vi "ConfigParseLoop.vi"(0 "Root Refnum in":refnum<k20>, 11 "error in (no error)":errorcluster) -> (4 "General Settings":string[][](array[string]), 6 "Loop Microscope Settings":string[][](array[string]), 8 "Position Settings":string[][](array[string]), 10 "Program":string[][](array[string]), 15 "error out":errorcluster)   [LabVIEW 2018, in "Config.lvlib"]
uses:
  Config.lvlib
  <vilib>/xml/NI_XML.lvlib
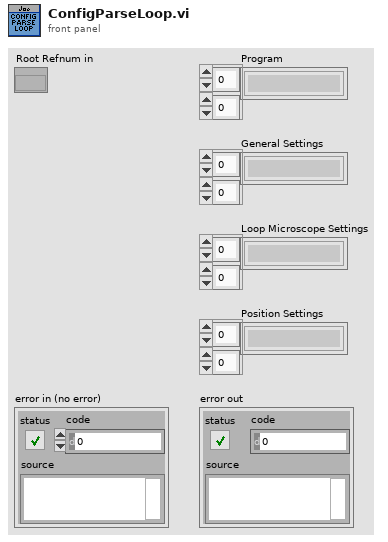
[diagram p1: front panel]
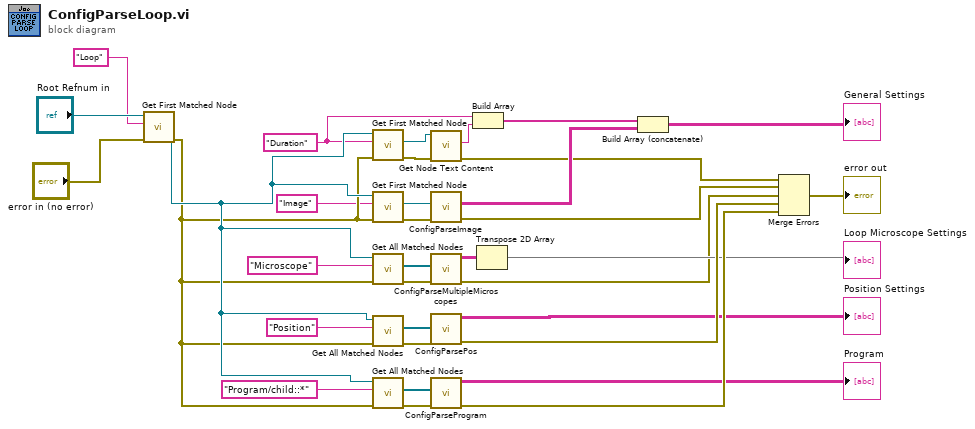
[diagram p0: block diagram]
diagram:
  w10 = "Duration" ("XPath expression")
  n1 = call <vilib>:"Get First Matched Node.vi"("error in (no error)"="error in (no error)", "XPath expression"="Loop" ("Get Elements By Tag Name"), "node in"="Root Refnum in") -> ("error out"=w22:errorcluster, "node result"=w24:refnum<k20>)  [unwired: 6 in, 1 out]
  n2 = call <vilib>:"Get First Matched Node.vi"("error in (no error)"=w22, "XPath expression"=w10, "node in"=w24) -> ("error out"=w11:errorcluster, "node result"=w8:refnum<k20>)  [unwired: 6 in, 1 out]
  n3 = call <vilib>:"Get First Matched Node.vi"("error in (no error)"=w22, "XPath expression"="Image", "node in"=w24) -> ("error out"=w12:errorcluster, "node result"=w25:refnum<k20>)  [unwired: 6 in, 1 out]
  n4 = call <vilib>:"Get All Matched Nodes.vi"("error in (no error)"=w22, "XPath expression"="Microscope", "node in"=w24) -> ("error out"=w13:errorcluster, "node result array"=w29:refnum<k20>[])  [unwired: 6 in, 1 out]
  n5 = call <vilib>:"Get All Matched Nodes.vi"("error in (no error)"=w22, "XPath expression"="Position", "node in"=w24) -> ("error out"=w6:errorcluster, "node result array"=w30:refnum<k20>[])  [unwired: 6 in, 1 out]
  n6 = call <vilib>:"Get All Matched Nodes.vi"("error in (no error)"=w22, "XPath expression"="Program/child::*", "node in"=w24) -> ("error out"=w21:errorcluster, "node result array"=w31:refnum<k20>[])  [unwired: 6 in, 1 out]
  n7 = call <vilib>:"Get Node Text Content.vi"("error in (no error)"=w11, "node in"=w8) -> ("error out"=w16:errorcluster, "node text"=w9:string)  [unwired: 7 in, 1 out]
  n8 = call "ConfigParseImage.vi"("error in (no error)"=w12, "Refnum in"=w25) -> ("error out"=w17:errorcluster, "Array out"=w27:string[][])  [unwired: 8 in]
  n9 = call "ConfigParseMultipleMicroscopes.vi"("error in (no error)"=w13, "node result array"=w29) -> ("error out"=w18:errorcluster, "Array"=w14:string[][])  [unwired: 8 in]
  n10 = call "ConfigParsePos.vi"("error in (no error)"=w6, "node result array"=w30) -> ("error out"=w20:errorcluster, "Array"=→"Position Settings":string[][])  [unwired: 8 in]
  n11 = call "ConfigParseProgram.vi"("error in (no error)"=w21, "node result array"=w31) -> ("error out"=w33:errorcluster, "Program Array"=→"Program":string[][])  [unwired: 8 in]
  n12 = Build Array(w10, w9) -> (w26:string[])
  n13 = Transpose 2D Array(2D array=w14) -> (transposed array=→"Loop Microscope Settings":string[][])
  n14 = Build Array (concatenate)(w26, w27) -> (→"General Settings":string[][])
  n15 = Merge Errors(w16, w17, w18, w20, w33) -> (→"error out":errorcluster)
